vi "Write WaitParams.vi"(8 "error in":errorcluster, 10 "WaitParams":cluster{"Timeout (ms)":u32, "LoopTime (ms)":u32}={"Timeout (ms)"=100, "LoopTime (ms)"=10}, 11 "Serial Session in":refnum<class "Serial Session.lvclass">) -> (0 "error out":errorcluster, 3 "Serial Session out":refnum<class "Serial Session.lvclass">)   [LabVIEW 2019, in "Serial Session.lvclass"]
doc: "Set the wait parameter property in the session. These will define how data will be retrieved from the port if the read does not terminate on a character."
uses:
  Serial Session.lvclass
  Serial Session.lvclass/Serial Session.ctl
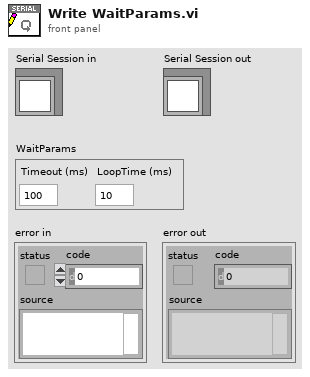
[diagram p1: front panel]
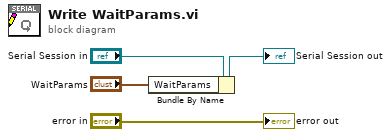
[diagram p0: block diagram]
diagram:
  n1 = Bundle By Name(cluster="Serial Session in", "WaitParams"="WaitParams") -> (→"Serial Session out":refnum<class "Serial Session.lvclass">)
  "error out" <- "error in"
